vi "Generate X Axis.vi"(1 "Axis Index":i32, 2 "Data Plot":T1) -> (0 "X Axis":dbl[](array[numeric]))   [LabVIEW 2019]
uses:
  Sub Controls/Data Graph.ctl
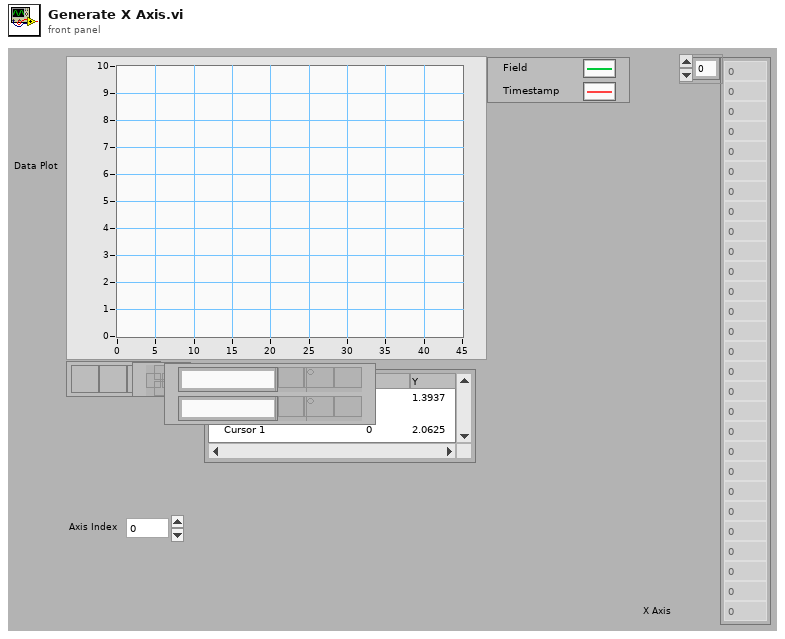
[diagram p1: front panel]
types:
  T1 = typedef "Data Graph.ctl" = cluster{dbl[], dbl[]}[]
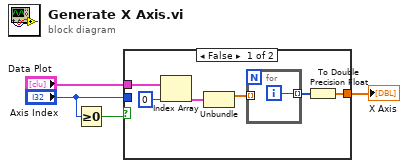
[diagram p0: block diagram]
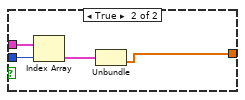
[diagram p2: hidden frame]
diagram:
  n1 = Greater Or Equal To 0?(x="Axis Index") -> (x >= 0?=w3:bool)
  n2 = case shown="False" w3 {
    tunnel: "Data Plot" -> [w9 w14]
    tunnel: [w5 w12] -> w2
    tunnel: "Axis Index" -> [_ w13]
    frame False {
      n3 = Index Array(array=w9, index=0) -> (element=w10:cluster{dbl[], dbl[]})
      n4 = Unbundle(w10) -> (w7:dbl[])  [unwired: 1 out]
      n5 = for {
        tunnel: w7 -> [_] mode=indexing
        tunnel: [w11] -> w6 mode=indexing
        i -> [w11]
      }
      n6 = To Double Precision Float(number=w6) -> (double precision float=w5:dbl[])
    }
    frame True {
      n7 = Index Array(array=w14, index=w13) -> (element=w15:cluster{dbl[], dbl[]})
      n8 = Unbundle(w15) -> (w12:dbl[])  [unwired: 1 out]
    }
  }
  "X Axis" <- w2
